vi "Enviar Iniciar Guardado.vi"(8 "error in (no error)":errorcluster, 10 "Save?":bool, 11 "Guardar TextoPlano in":refnum<class "Guardar TextoPlano.lvclass">) -> (0 "error out":errorcluster, 3 "Guardar TextoPlano out":refnum<class "Guardar TextoPlano.lvclass">)   [LabVIEW 2020, in "Guardar TextoPlano.lvlib" / "Guardar TextoPlano.lvclass"]
uses:
  Guardar TextoPlano.lvclass
  Guardar TextoPlano.lvclass/Guardar TextoPlano.ctl
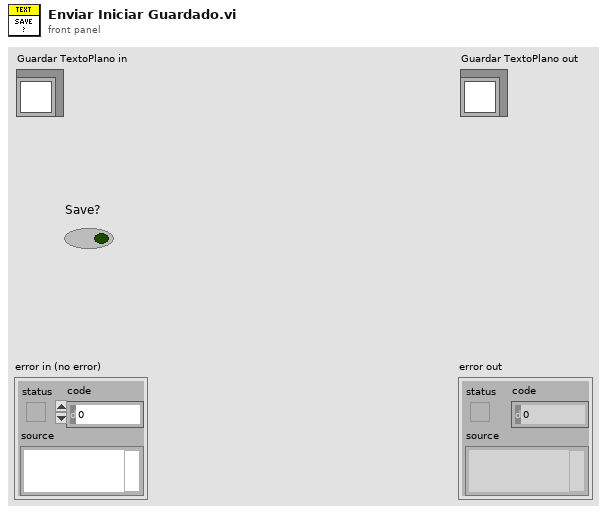
[diagram p1: front panel]
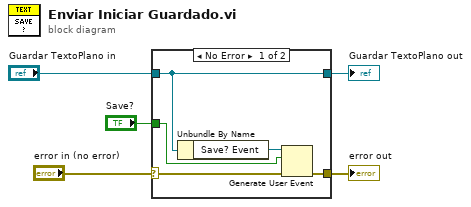
[diagram p0: block diagram]
diagram:
  n1 = case shown="No Error" "error in (no error)" {
    selector: "error in (no error)" -> [w9 w12]
    tunnel: [w8 w12] -> w4
    tunnel: [w10 w11] -> w2
    tunnel: "Guardar TextoPlano in" -> [w10 w11]
    tunnel: "Save?" -> [w6 _]
    frame No Error {
      n2 = Unbundle By Name(w10) -> ("Save? Event"=w7:refnum<user-event>)
      n3 = Generate User Event(user event=w7, event data cluster=w6, error in=w9) -> (error out=w8:errorcluster)  [unwired: 1 in, 1 out]
    }
    frame Error {
    }
  }
  "error out" <- w4
  "Guardar TextoPlano out" <- w2
